vi "Read Sample from Container.vi"(8 "error in (no error)":errorcluster, 10 "Container":T1, 11 "Storage Line in":refnum<class "Storage Line.lvclass">) -> (0 "error out":errorcluster, 2 "Sample":refnum<class "Sample.lvclass">, 3 "Storage Line out":refnum<class "Storage Line.lvclass">)   [LabVIEW 2015, in "cRIO-Carbondioxide.lvlib" / "CO2-Actor.lvlib" / "Storage Line.lvclass"]
uses:
  Storage Line.lvclass
  Controls/Sample Transfer Container Enumerator.ctl
  subs/Sample/Sample.lvclass
  Storage Line.lvclass/Storage Line.ctl
  CO2 Actor/CO2 Actor.lvclass
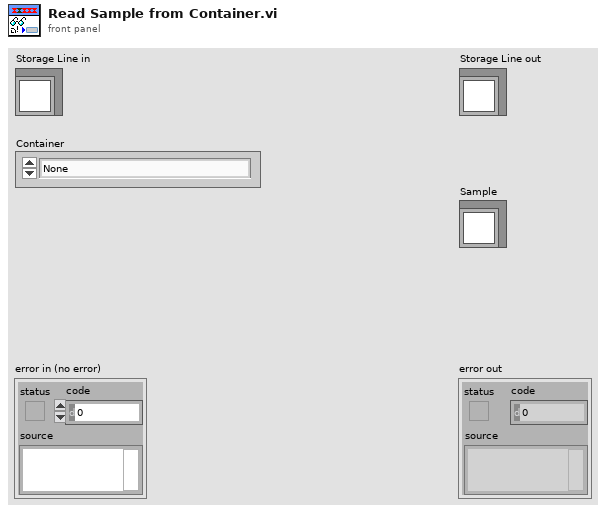
[diagram p1: front panel]
types:
  T1 = typedef "Sample Transfer Container Enumerator.ctl" = enum16{"None", "Sample 1", "Sample 2", "Sample 3", "Sample 4", "Sample 5", "Storage 01", "Storage 02", "Storage 03", "Storage 04", "Storage 05", "Storage 06", "Storage 07", "Storage 08", "Storage 09", "Storage 10", "Storage 11", "Storage 12", "Syringe", "Undefined"}
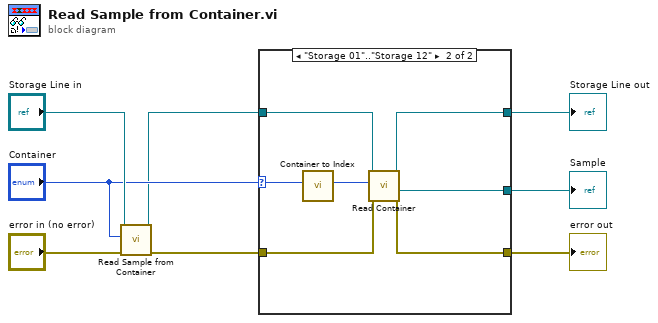
[diagram p0: block diagram]
diagram:
  n1 = call-parent "Read Sample from Container.vi"("error in (no error)"="error in (no error)", "Container"="Container", "CO2 Actor in"="Storage Line in") -> ("error out"=w3:errorcluster, "CO2 Actor out"=w4:refnum<class "Storage Line.lvclass">)  [unwired: 6 in, 1 out]
  n2 = case shown="\"Storage 01\"..\"Storage 12\"" "Container" {
    selector: "Container" -> [_ w17]
    tunnel: [w10 w15] -> w5
    tunnel: w4 -> [w10 w16]
    tunnel: w3 -> [w9 w12]
    tunnel: [w9 w11] -> w2
    tunnel: [_ w13] -> w1
    frame "None", Default {
    }
    frame "Storage 01".."Storage 12" {
      n3 = call "Container to Index.vi"("Container"=w17) -> ("Index"=w14:i32)  [unwired: 10 in]
      n4 = call "Read Container.vi"("error in (no error)"=w12, "index"=w14, "Storage Line in"=w16) -> ("error out"=w11:errorcluster, "Sample out"=w13:refnum<class "Sample.lvclass">, "Storage Line out"=w15:refnum<class "Storage Line.lvclass">)  [unwired: 5 in, 1 out]
    }
  }
  "error out" <- w2
  "Storage Line out" <- w5
  "Sample" <- w1
